vi "ziGetCurrentCalc.vi"   [LabVIEW 2009, in "Zurich Instruments LabOne.lvlib"]
uses:
  <instrlib>/Zurich Instruments LabOne/Zurich Instruments LabOne.lvlib
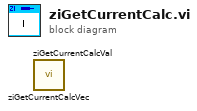
[diagram p0: block diagram]
diagram:
  n1 = call <instrlib>:"ziGetCurrentCalcVec.vi"() -> ()  [unwired: 11 in, 1 out]
  n2 = call <instrlib>:"ziGetCurrentCalcVal.vi"() -> ()  [unwired: 11 in, 1 out]
